vi "Add File.vi"(8 "error in (no error)":errorcluster, 9 "Insert in front":bool=TRUE, 10 "File Path":path, 11 "XY WFRM Plot in":refnum<class "XY WFRM Plot.lvclass">) -> (0 "error out":errorcluster, 2 "Success":bool, 3 "XY WFRM Plot out":refnum<class "XY WFRM Plot.lvclass">)   [LabVIEW 2015, in "XY WFRM Plot.lvclass"]
uses:
  XY WFRM Plot.lvclass
  XY WFRM Plot.lvclass/XY WFRM Plot.ctl
  Plot/Plot.lvclass/Plot.ctl
  Read Files ref.vi
  Plot/Read Files.vi
  Read X column ref.vi
  Read Y columns ref.vi
  Plot/Plot.lvclass
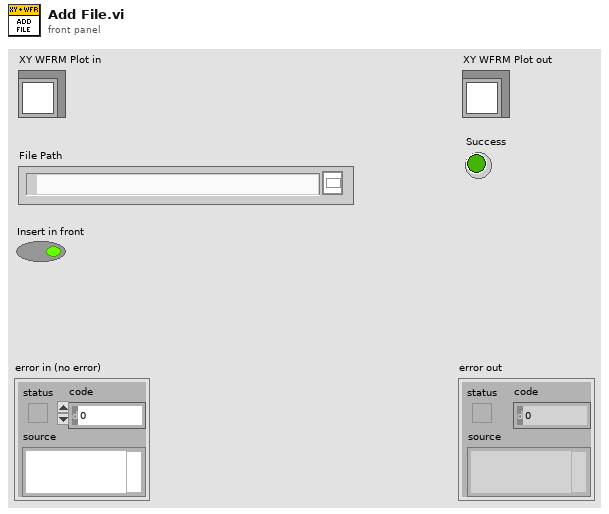
[diagram p1: front panel]
types:
  T1 = typedef "File_Group_Chan_Abbr.ctl" = cluster{"File Path Control":path, "Group":string, "Channel":string, "Abbreviated":string}
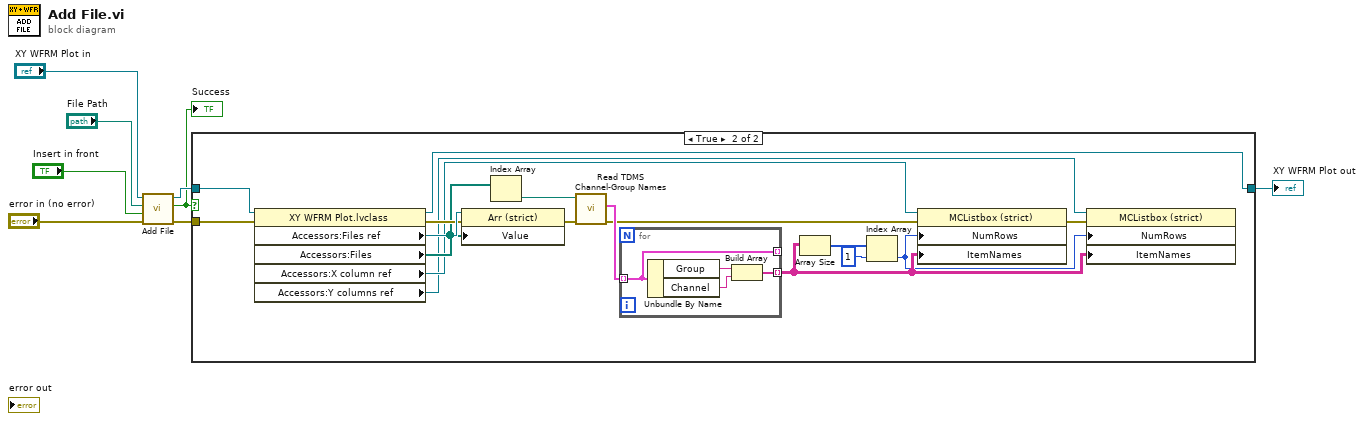
[diagram p0: block diagram]
diagram:
  n1 = call-parent "Add File.vi"("error in (no error)"="error in (no error)", "Insert in front"="Insert in front", "File Path"="File Path", "Plot in"="XY WFRM Plot in") -> ("error out"=w2:errorcluster, "Success"=w1:bool, "Plot out"=w8:refnum<class "XY WFRM Plot.lvclass">)  [unwired: 5 in]
  "Success" <- w1
  n2 = case shown="True" w1 {
    tunnel: w8 -> [w9 w26]
    tunnel: [w9 w25] -> w3
    tunnel: w2 -> [_ w24]
    frame False {
    }
    frame True {
      n3 = property class="XY WFRM Plot.lvclass"(reference=w26, error in=w24) -> (reference out=w25:refnum<class "XY WFRM Plot.lvclass">, error out=w22:errorcluster, "Accessors:Files ref"=w23:refnum<vi>, "Accessors:Files"=w21:path[], "Accessors:X column ref"=w17:refnum<vi>, "Accessors:Y columns ref"=w16:refnum<vi>)
      n4 = property class="Arr (strict)"(reference=w23, error in=w22, "Value"=w21) -> (error out=w19:errorcluster)  [unwired: 1 out]
      n5 = Index Array(array=w21) -> (element=w20:path)  [unwired: 1 in]
      n6 = call "Read TDMS Channel-Group Names.vi"("error in"=w19, "File Path Control"=w20) -> ("error out"=w15:errorcluster, "File-group-channel"=w18:T1[])  [unwired: 8 in]
      n7 = for {
        tunnel: [w30] -> _ mode=indexing
        tunnel: w18 -> [w30] mode=indexing
        tunnel: [w27] -> w11 mode=indexing
        n8 = Unbundle By Name(w30) -> ("Group"=w29:string, "Channel"=w28:string)
        n9 = Build Array(w29, w28) -> (w27:string[])
      }
      n10 = Array Size(array=w11) -> (size(s)=w13:i32[])
      n11 = Index Array(array=w13, index=1) -> (element=w10:i32)
      n12 = property class="MCListbox (strict)"(reference=w17, error in=w15, "NumRows"=w10, "ItemNames"=w11) -> (error out=w14:errorcluster)  [unwired: 1 out]
      n13 = property class="MCListbox (strict)"(reference=w16, error in=w14, "NumRows"=w10, "ItemNames"=w11) -> ()  [unwired: 2 out]
    }
  }
  "XY WFRM Plot out" <- w3
